vi "vision data fg.vi"(1 "Input":T1, 2 "Menu":T2) -> (0 "Output":T1)   [LabVIEW 2014]
uses:
  typedefs/fg_getset.ctl
  typedefs/vision/vision data.ctl
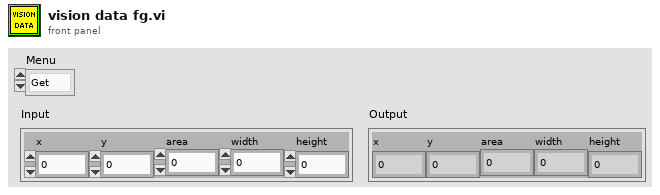
[diagram p1: front panel]
types:
  T1 = typedef "vision data.ctl" = cluster{"x":dbl, "y":dbl, "area":dbl, "width":dbl, "height":dbl}
  T2 = typedef "fg_getset.ctl" = enum16{"Get", "Set"}
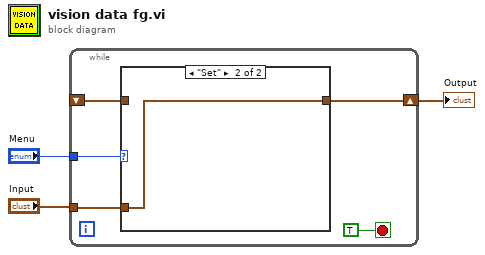
[diagram p0: block diagram]
diagram:
  n1 = while {
    shift-right: [w5] -> w3
    shift-left: _ -> [w7]
    tunnel: "Input" -> [w6]
    tunnel: "Menu" -> [w4]
    stop <- TRUE stop-if-true
    n2 = case shown="\"Set\"" w4 {
      tunnel: w7 -> [w9 _]
      tunnel: w6 -> [_ w10]
      tunnel: [w9 w10] -> w5
      frame "Get", Default {
      }
      frame "Set" {
      }
    }
  }
  "Output" <- w3
